vi "Queue_Driver.vi"(0 "State_In":string, 2 "Queue_Name_In":string, 5 "N_State_In":string[](array[string]), 7 "Time_Out_In_ms (10)":i32=10, 9 "Max_Queue_Size_In":i32=-1, 11 "Error_In":errorcluster, 13 "Queue_Operation_Select":T1=enum."Flush") -> (4 "State_Out":string, 15 "Error_Out":errorcluster)   [LabVIEW 2021]
doc: "Used to send the states data from one loop to another."
uses:
  Controls/Queue_Operation_Select.ctl
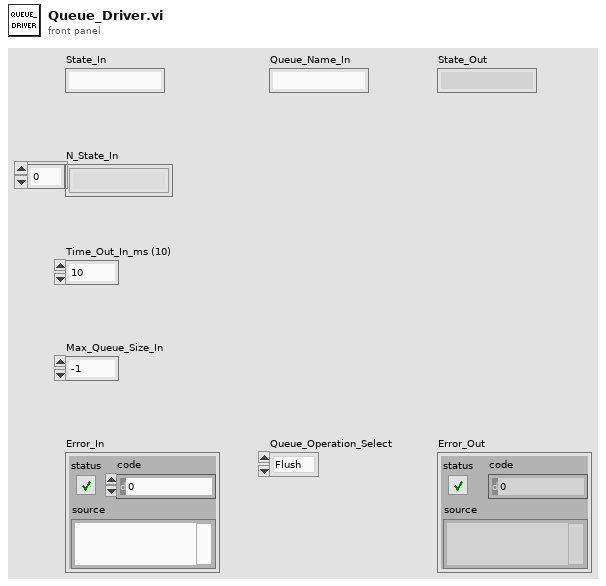
[diagram p1: front panel]
types:
  T1 = typedef "Queue_Operation_Select.ctl" = enum16{"Obtain_Queue", "Enqueue", "Enqueue_N", "Enqueue_at_End", "Dequeue", "Flush", "Release_Queue"}
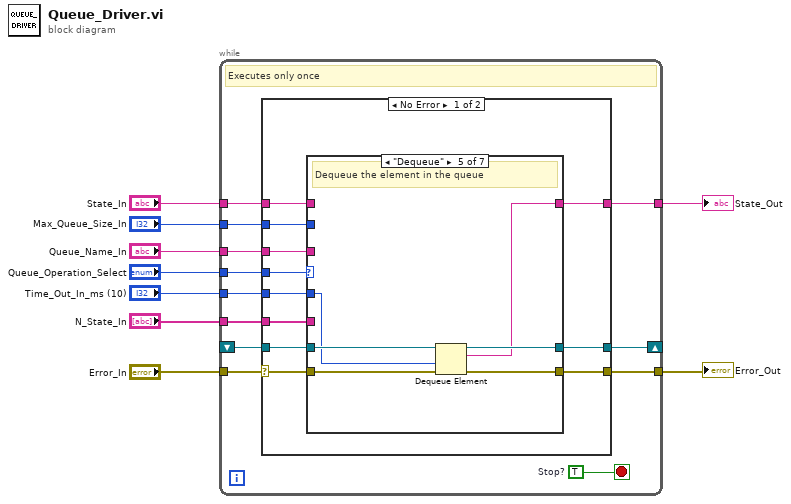
[diagram p0: block diagram]
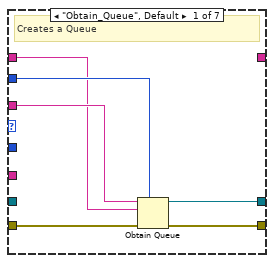
[diagram p2: hidden frame]
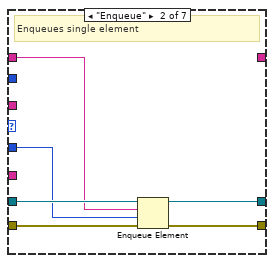
[diagram p3: hidden frame]
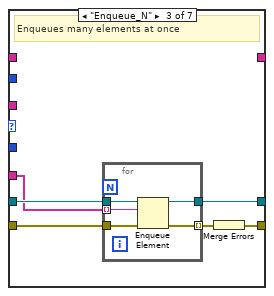
[diagram p4: hidden frame]
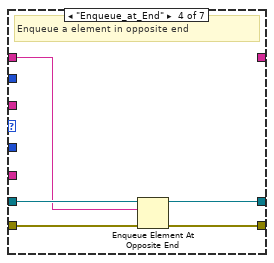
[diagram p5: hidden frame]
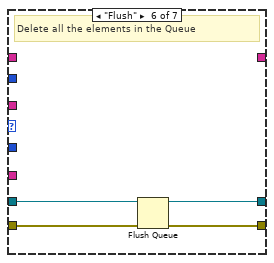
[diagram p6: hidden frame]
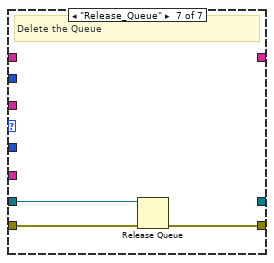
[diagram p7: hidden frame]
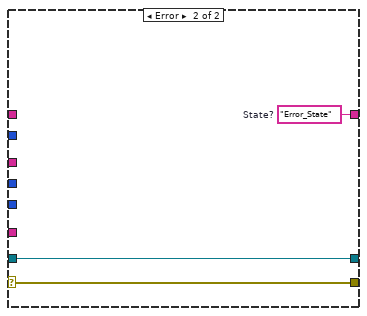
[diagram p8: hidden frame]
diagram:
  n1 = while {
    tunnel: "Error_In" -> [w21]
    tunnel: "N_State_In" -> [w20]
    tunnel: "Time_Out_In_ms (10)" -> [w19]
    tunnel: "Queue_Operation_Select" -> [w18]
    tunnel: "Queue_Name_In" -> [w17]
    tunnel: "Max_Queue_Size_In" -> [w16]
    tunnel: "State_In" -> [w15]
    tunnel: [w14] -> w2
    tunnel: [w13] -> w1
    shift-right: [w11] -> _
    shift-left: _ -> [w12]
    stop <- w10 stop-if-true
    w10 = TRUE  # Stop?
    # "Executes only once"
    n2 = case shown="No Error" w21 {
      selector: w21 -> [w32 w76]
      tunnel: w20 -> [w31 _]
      tunnel: w19 -> [w30 _]
      tunnel: w18 -> [w29 _]
      tunnel: w17 -> [w28 _]
      tunnel: w16 -> [w27 _]
      tunnel: w15 -> [w26 _]
      tunnel: [w25 w74] -> w14
      tunnel: [w24 w76] -> w13
      tunnel: w12 -> [w23 w75]
      tunnel: [w22 w75] -> w11
      frame No Error {
        n3 = case shown="\"Dequeue\"" w29 {
          tunnel: w32 -> [w38 w44 w46 w59 w65 w69 w72]
          tunnel: w28 -> [w36 _ _ _ _ _ _]
          tunnel: w27 -> [w35 _ _ _ _ _ _]
          tunnel: [w33 w40 w49 w58 w64 w68 _] -> w22
          tunnel: [w37 w43 w45 w57 w62 w67 w71] -> w24
          tunnel: w23 -> [_ w42 w50 w60 w66 w70 w73]
          tunnel: w26 -> [w34 w41 _ w56 _ _ _]
          tunnel: w30 -> [_ w39 _ _ w61 _ _]
          tunnel: [_ _ _ _ w63 _ _] -> w25
          tunnel: w31 -> [_ _ w47 _ _ _ _]
          frame "Obtain_Queue", Default {
            # "Creates a Queue"
            n4 = Obtain Queue(max queue size (-1, unlimited)=w35, name (unnamed)=w36, element data type=w34, error in (no error)=w38) -> (queue out=w33:refnum<queue>, error out=w37:errorcluster)  [unwired: 1 in, 1 out]
          }
          frame "Enqueue" {
            # "Enqueues single element"
            n5 = Enqueue Element(queue=w42, element=w41, timeout in ms (-1)=w39, error in (no error)=w44) -> (queue out=w40:refnum<queue>, error out=w43:errorcluster)  [unwired: 1 out]
          }
          frame "Enqueue_N" {
            # "Enqueues many elements at once"
            n6 = for {
              tunnel: w50 -> [w55]
              tunnel: [w53] -> w49
              tunnel: w47 -> [w51] mode=indexing
              tunnel: w46 -> [w54]
              tunnel: [w52] -> w48 mode=indexing
              n7 = Enqueue Element(queue=w55, element=w51, error in (no error)=w54) -> (queue out=w53:refnum<queue>, error out=w52:errorcluster)  [unwired: 1 in, 1 out]
            }
            n8 = Merge Errors(w48) -> (w45:errorcluster)
          }
          frame "Enqueue_at_End" {
            # "Enqueue a element in opposite end"
            n9 = Enqueue Element At Opposite End(queue=w60, element=w56, error in (no error)=w59) -> (queue out=w58:refnum<queue>, error out=w57:errorcluster)  [unwired: 1 in, 1 out]
          }
          frame "Dequeue" {
            # "Dequeue the element in the queue"
            n10 = Dequeue Element(queue=w66, timeout in ms (-1)=w61, error in (no error)=w65) -> (queue out=w64:refnum<queue>, element=w63:string, error out=w62:errorcluster)  [unwired: 1 out]
          }
          frame "Flush" {
            # "Delete all the elements in the Queue"
            n11 = Flush Queue(queue=w70, error in (no error)=w69) -> (queue out=w68:refnum<queue>, error out=w67:errorcluster)  [unwired: 1 out]
          }
          frame "Release_Queue" {
            # "Delete the Queue"
            n12 = Release Queue(queue=w73, error in (no error)=w72) -> (error out=w71:errorcluster)  [unwired: 1 in, 2 out]
          }
        }
      }
      frame Error {
        w74 = "Error_State"  # State?
      }
    }
  }
  "Error_Out" <- w1
  "State_Out" <- w2
